vi "FPGA_Communication.vi"() -> ()   [LabVIEW 2020]
uses:
  <vilib>/rvi/interface/nirviMethod/nirviMethod.xnode
  <vilib>/FPGAPlugInAG/Dynamic/niLvFpga_Run_Dynamic.vi
  <vilib>/rvi/interface/nirviOpenFPGA/nirviOpenFPGA.xnode
  <vilib>/rvi/interface/nirviCloseFPGA/nirviCloseFPGA.xnode
  <vilib>/FPGAPlugInAG/Dynamic/niLvFpga_Close_Dynamic.vi
  <vilib>/FPGAPlugInAG/Dynamic/niLvFpga_ReadFifo_Dynamic.vi
  <vilib>/rvi/errors/niLvFpgaMergeErrorWithErrorCode.vi
  <vilib>/FPGAPlugInAG/Dynamic/niLvFpga_WriteFifo_Dynamic.vi
  FPGA Bitfiles/recog_FPGATarget_FPGA-code_DAMpIhrRJnA.lvbitx
  ANN/FPGA-code.vi
  <vilib>/FPGAPlugInAG/IC-3173/niLvFpga_Open_IC-3173.vi
  <vilib>/rvi/interface/common/dynamic/niFpgaDynamicAddResources.vi
panel:
  in  "stop":bool
  out "Data":bool[](array[boolean])
  out "Sended":sgl[](array[numeric])
  out "Received":sgl[](array[numeric])
  out "error out":errorcluster
  out "# elements":u32
  out "empty?":bool
  out "Intial Bias\n& Weights 2":dbl[](array[numeric])
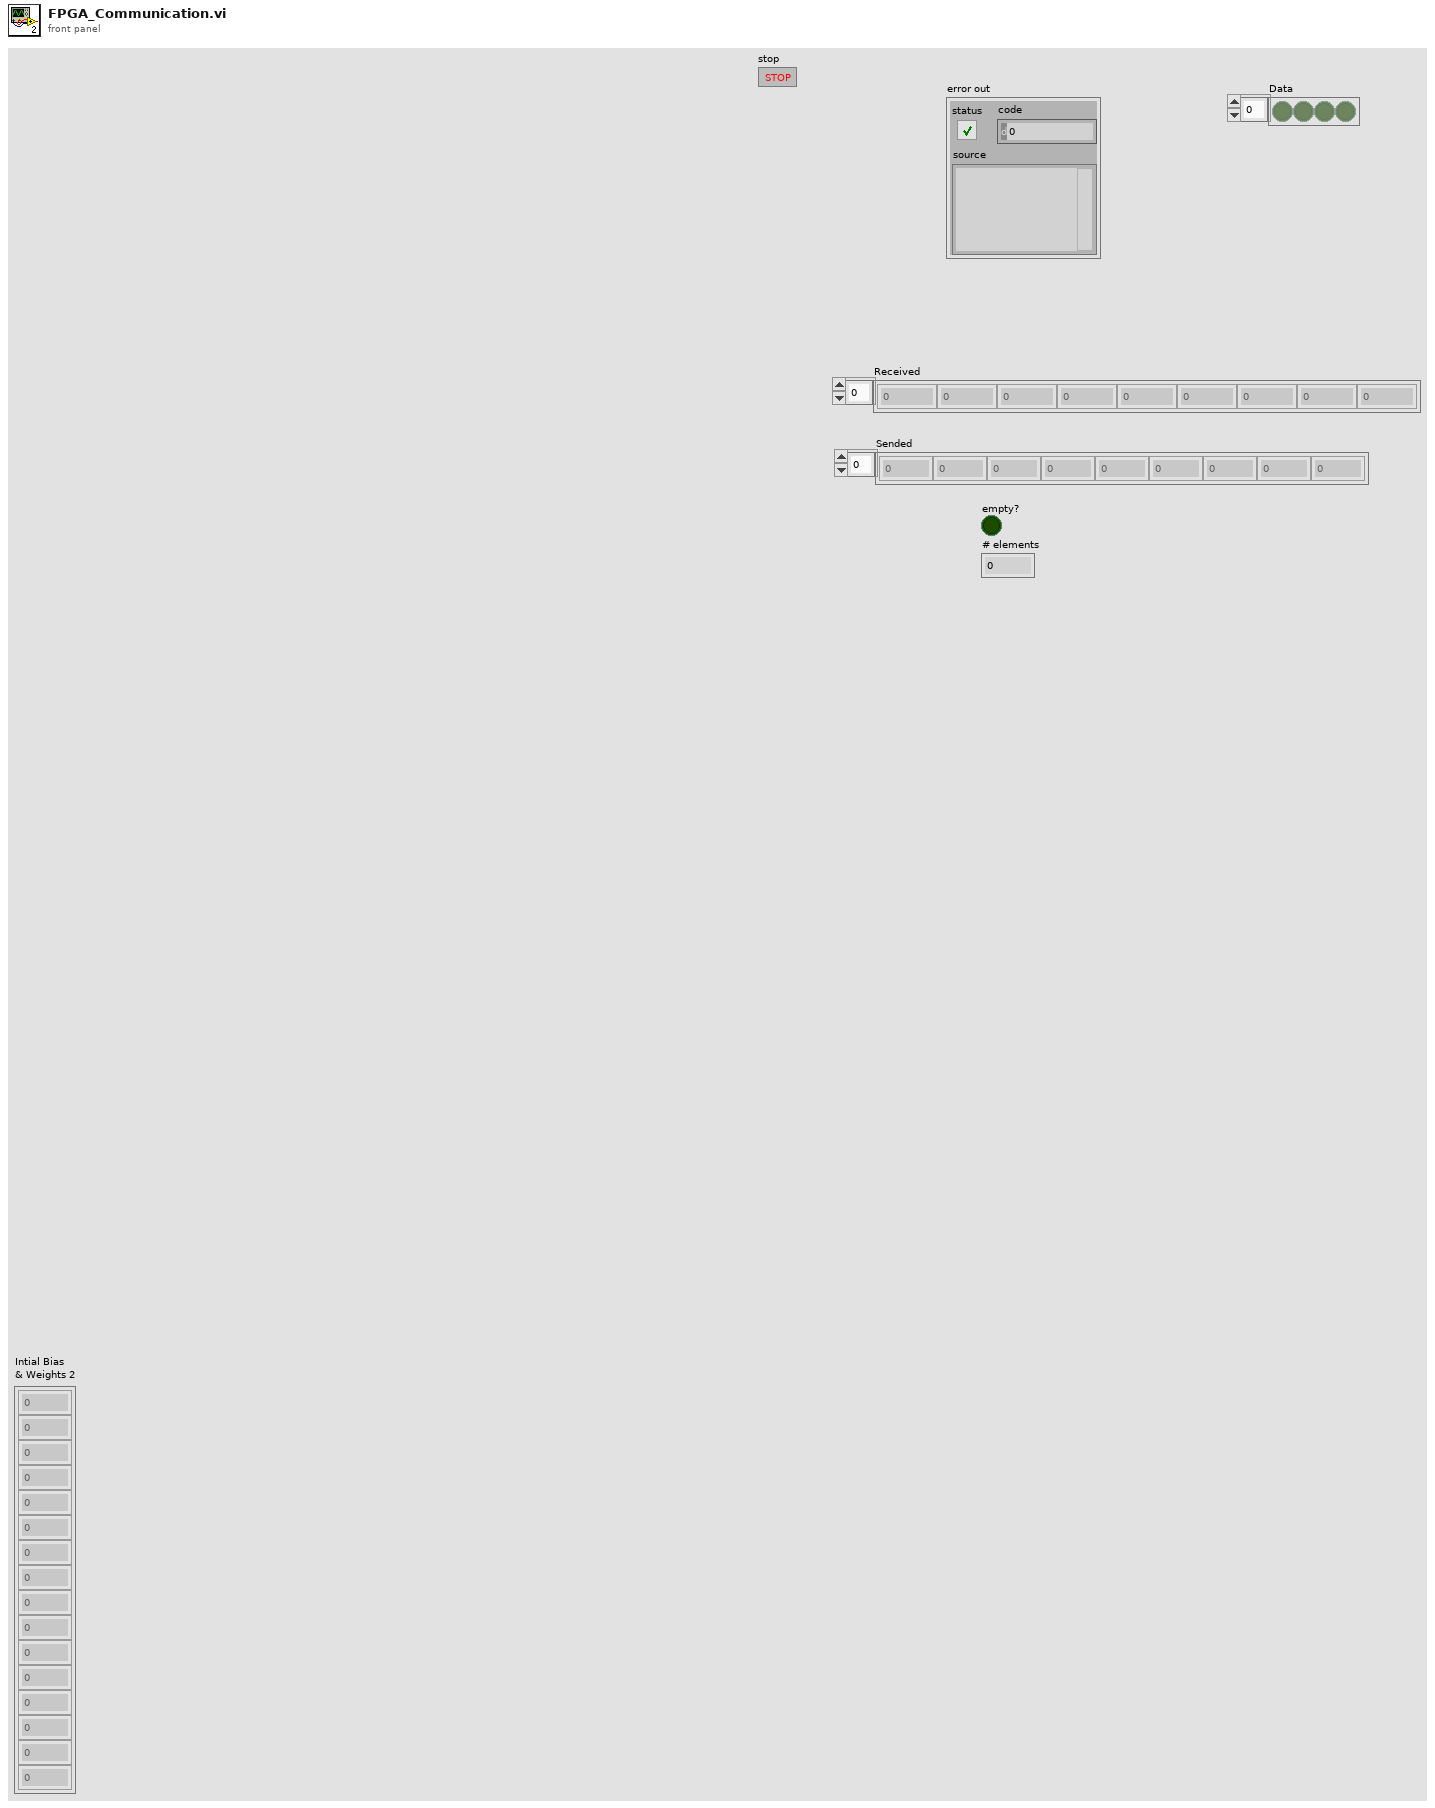
[diagram p1: front panel]
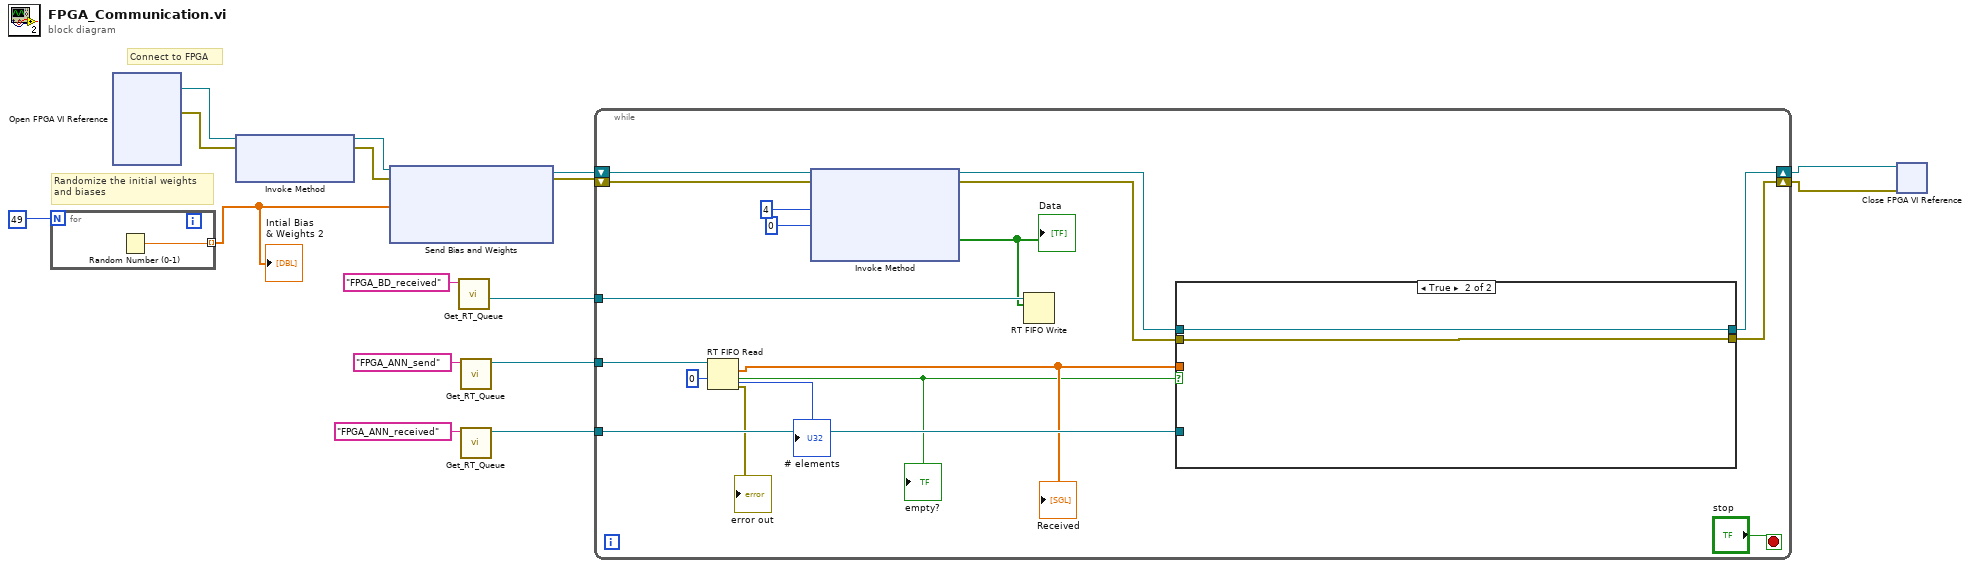
[diagram p0: block diagram]
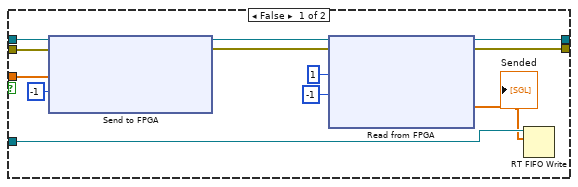
[diagram p2: hidden frame]
diagram:
  # "Randomize the initial weights \nand biases"
  # "Connect to FPGA"
  n1 = for {
    N: 49 -> [_]
    tunnel: [w17] -> w1 mode=indexing
    n2 = Random Number (0-1)() -> (number: 0 to 1=w17:dbl)
  }
  "Intial Bias\n& Weights 2" <- w1
  n3 = xnode "Open FPGA VI Reference"() -> ("FPGA VI Reference Out"=w12:refnum<k20>, "error out"=w13:errorcluster)  [unwired: 2 in]
  n4 = xnode "Invoke Method"("FPGA VI Reference In"=w12, "error in"=w13) -> ("FPGA VI Reference Out"=w3:refnum<k20>, "error out"=w2:errorcluster)  [unwired: 1 in]
  n5 = xnode "Send Bias and Weights"("FPGA VI Reference In"=w3, "error in"=w2, "Data"=w1) -> ("FPGA VI Reference Out"=w5:refnum<k20>, "error out"=w4:errorcluster)  [unwired: 1 in, 1 out]
  n6 = call "Get_RT_Queue.vi"("String"="FPGA_BD_received") -> ("rt fifo boolean"=w9:refnum<k33>)  [unwired: 8 in, 2 out]
  n7 = call "Get_RT_Queue.vi"("String"="FPGA_ANN_send") -> ("rt fifo single"=w8:refnum<k33>)  [unwired: 8 in, 2 out]
  n8 = call "Get_RT_Queue.vi"("String"="FPGA_ANN_received") -> ("rt fifo single"=w7:refnum<k33>)  [unwired: 8 in, 2 out]
  n9 = while {
    shift-right: [w24] -> w10
    shift-left: w4 -> [w32]
    shift-right: [w25] -> w11
    shift-left: w5 -> [w33]
    tunnel: w9 -> [w31]
    tunnel: w8 -> [w29]
    tunnel: w7 -> [w28]
    stop <- "stop" stop-if-true
    n10 = RT FIFO Read(0:w29, 2:0 ("timeout in ms (0)")) -> (7:→"# elements":u32, 9:w23:sgl[], 10:w21:bool, 11:→"error out":errorcluster)  [unwired: 2 in, 1 out]
    "empty?" <- w21
    "Received" <- w23
    n11 = xnode "Invoke Method"("FPGA VI Reference In"=w33, "error in"=w32, "Number of Elements"=4, "Timeout (ms)"=0) -> ("FPGA VI Reference Out"=w27:refnum<k20>, "error out"=w26:errorcluster, "Data"=w30:bool[])  [unwired: 1 out]
    "Data" <- w30
    n12 = RT FIFO Write(0:w31, 1:w30) -> ()  [unwired: 3 in, 4 out]
    n13 = case shown="True" w21 {
      tunnel: w28 -> [w39 _]
      tunnel: w27 -> [w43 w49]
      tunnel: w26 -> [w42 w48]
      tunnel: [w41 w49] -> w25
      tunnel: [w40 w48] -> w24
      tunnel: w23 -> [w37 _]
      frame False {
        n14 = xnode "Send to FPGA"("FPGA VI Reference In"=w43, "error in"=w42, "Data"=w37, "Timeout (ms)"=-1) -> ("FPGA VI Reference Out"=w46:refnum<k20>, "error out"=w45:errorcluster)  [unwired: 1 out]
        n15 = xnode "Read from FPGA"("FPGA VI Reference In"=w46, "error in"=w45, "Number of Elements"=u32 1, "Timeout (ms)"=-1 ("Number of Elements")) -> ("FPGA VI Reference Out"=w41:refnum<k20>, "error out"=w40:errorcluster, "Data"=w38:sgl[])  [unwired: 1 out]
        "Sended" <- w38
        n16 = RT FIFO Write(0:w39, 1:w38) -> ()  [unwired: 3 in, 4 out]
      }
      frame True {
      }
    }
  }
  n17 = xnode "Close FPGA VI Reference"("FPGA VI Reference In"=w11, "error in"=w10) -> ()  [unwired: 1 out]
